vi "NF WF1973_74 VOLT Rang.vi"(6 "Read(F)":bool, 8 "error in (no error)":errorcluster caption="Error IN", 9 "Auto Range(ON)":bool=TRUE, 10 "Ch(Ch1)":bool, 11 "VISAsession":refnum<visa-resource-name>) -> (0 "error out":errorcluster caption="Error OUT", 2 "Query Auto Range":string, 3 "CopyVISAsession":refnum<visa-resource-name>)   [LabVIEW 2010]
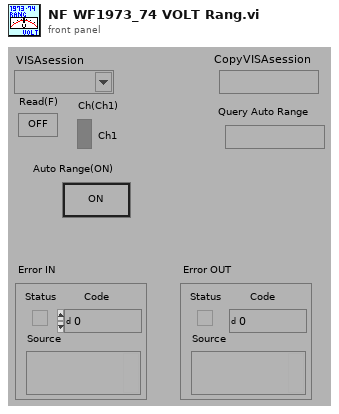
[diagram p1: front panel]
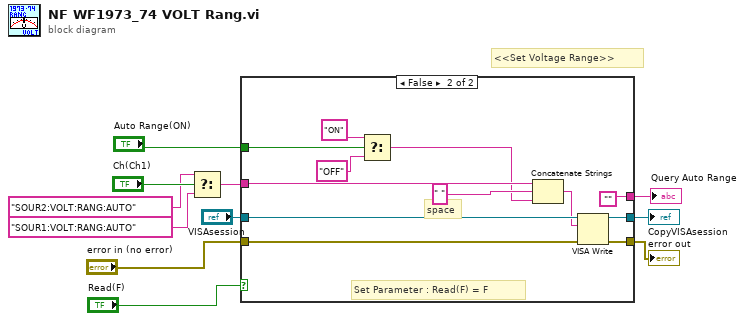
[diagram p0: block diagram]
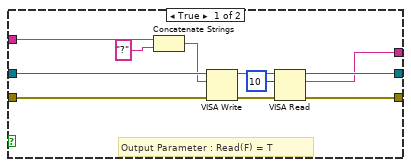
[diagram p2: hidden frame]
diagram:
  # "<<Set Voltage Range>>"
  n1 = Select(t="SOUR2:VOLT:RANG:AUTO" ("文字列"), s="Ch(Ch1)", f="SOUR1:VOLT:RANG:AUTO" ("文字列")) -> (s? t:f=w4:string)
  n2 = case shown="FALSE" "Read(F)" {
    tunnel: "VISAsession" -> [w22 w34]
    tunnel: [w19 w32] -> w10
    tunnel: [w18 w33] -> w9
    tunnel: "error in (no error)" -> [w17 w28]
    tunnel: w4 -> [w15 w29]
    tunnel: [w12 ""] -> w6
    tunnel: "Auto Range(ON)" -> [_ w24]
    frame True {
      # "Output Parameter : Read(F) = T"
      n3 = Concatenate Strings(w15, "?" ("形式文字列")) -> (w13:string)
      n4 = VISA Write(VISA resource name=w22, write buffer=w13, error in (no error)=w17) -> (VISA resource name out=w20:refnum<visa-resource-name>, error out=w21:errorcluster)  [unwired: 1 out]
      n5 = VISA Read(VISA resource name=w20, byte count=u32 10 ("バイトカウント（0）"), error in (no error)=w21) -> (VISA resource name out=w19:refnum<visa-resource-name>, read buffer=w12:string, error out=w18:errorcluster)  [unwired: 1 out]
    }
    frame False {
      # "space"
      # "Set Parameter : Read(F) = F"
      n6 = Select(t="ON", s=w24, f="OFF") -> (s? t:f=w23:string)
      n7 = Concatenate Strings(w29, " ", w23) -> (w31:string)
      n8 = VISA Write(VISA resource name=w34, write buffer=w31, error in (no error)=w28) -> (VISA resource name out=w32:refnum<visa-resource-name>, error out=w33:errorcluster)  [unwired: 1 out]
    }
  }
  "error out" <- w9
  "CopyVISAsession" <- w10
  "Query Auto Range" <- w6
